vi "Add Hierarchy to Tree.vi"(7 "file name":string, 8 "error in":errorcluster, 10 "file contents":cluster{"group":string, "channels":string[]}[](array[cluster]), 11 "file tree refnum":refnum<vi>) -> (0 "error out":errorcluster)   [LabVIEW 2020, in "TdmsFileViewer.lvlib"]
uses:
  TdmsFileViewer.lvlib
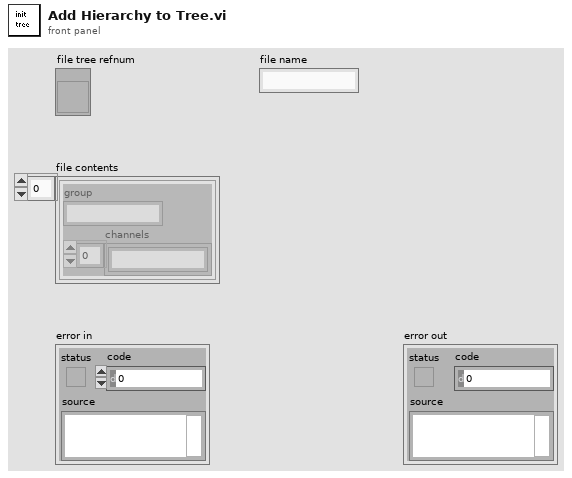
[diagram p1: front panel]
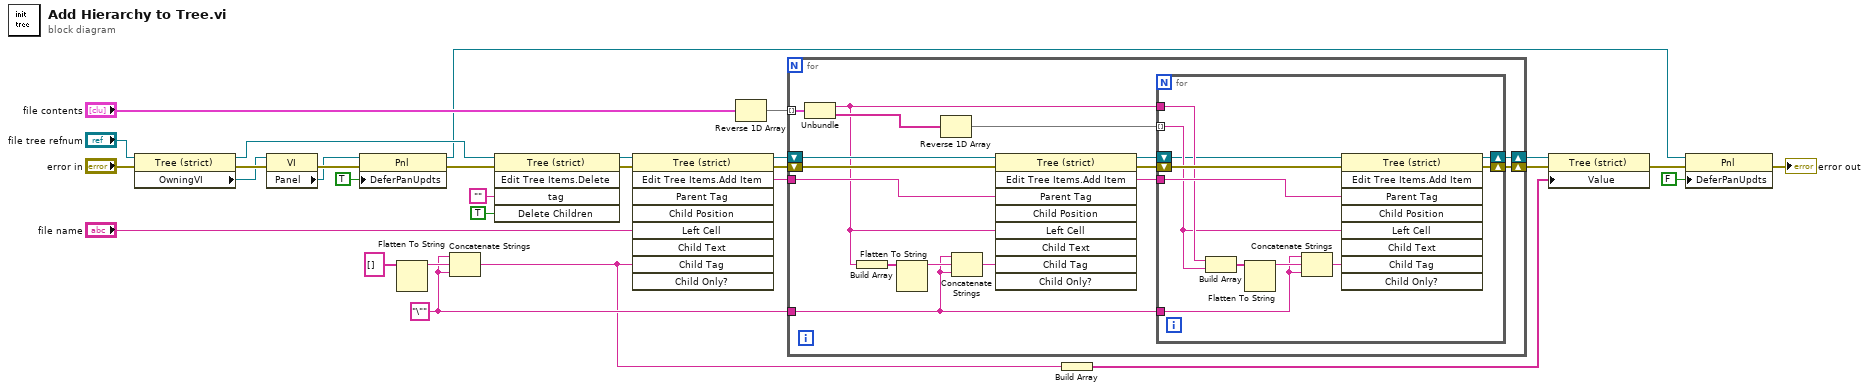
[diagram p0: block diagram]
diagram:
  w15 = "\"" ("string")
  n1 = property class="Tree (strict)"(reference="file tree refnum", error in="error in") -> (reference out=w6:refnum<vi>, error out=w26:errorcluster, "OwningVI"=w8:refnum<vi>)
  n2 = property class="VI"(reference=w8, error in=w26) -> (error out=w25:errorcluster, "Panel"=w7:refnum<vi>)  [unwired: 1 out]
  n3 = property class="Pnl"(reference=w7, error in=w25, "DeferPanUpdts"=TRUE ("Defer Panel Updates")) -> (reference out=w3:refnum<vi>, error out=w24:errorcluster)
  n4 = Flatten To String(anything=string[] [] ("appended array")) -> (data string=w18:string)  [unwired: 3 in, 2 out]
  n5 = Concatenate Strings(w15, w18, w15) -> (w2:string)
  n6 = invoke on="Invoke Node" class="Tree (strict)" method="Edit Tree Items.Delete"(reference=w6, error in=w24, "tag"="" ("Tag"), "Delete Children"=TRUE ("Delete Children?")) -> (reference out=w13:refnum<vi>, error out=w29:errorcluster)  [unwired: 1 in, 3 out]
  n7 = invoke on="Invoke Node" class="Tree (strict)" method="Edit Tree Items.Add Item"(reference=w13, error in=w29, "Left Cell"="file name", "Child Tag"=w2) -> (reference out=w20:refnum<vi>, error out=w30:errorcluster, "Edit Tree Items:Add Item"=w16:string)  [unwired: 5 in, 6 out]
  n8 = Reverse 1D Array(array="file contents") -> (reversed array=w21:cluster{"group":string, "channels":string[]}[])
  n9 = for {
    tunnel: w21 -> [w34] mode=indexing
    shift-right: [w45] -> w28
    shift-left: w30 -> [w46]
    tunnel: w16 -> [w42]
    tunnel: w15 -> [w35]
    shift-right: [w31] -> w10
    shift-left: w20 -> [w43]
    n10 = Unbundle(w34) -> ("group"=w32:string, "channels"=w33:string[])
    n11 = Build Array(w32) -> (w40:string[])
    n12 = Flatten To String(anything=w40) -> (data string=w38:string)  [unwired: 3 in, 2 out]
    n13 = Reverse 1D Array(array=w33) -> (reversed array=w39:string[])
    n14 = Concatenate Strings(w35, w38, w35) -> (w37:string)
    n15 = invoke on="Invoke Node" class="Tree (strict)" method="Edit Tree Items.Add Item"(reference=w43, error in=w46, "Parent Tag"=w42, "Left Cell"=w32, "Child Tag"=w37) -> (reference out=w36:refnum<vi>, error out=w44:errorcluster, "Edit Tree Items:Add Item"=w41:string)  [unwired: 4 in, 6 out]
    n16 = for {
      tunnel: w39 -> [w53] mode=indexing
      shift-right: [w56] -> w45
      shift-left: w44 -> [w57]
      tunnel: w41 -> [w55]
      tunnel: w32 -> [w54]
      tunnel: w35 -> [w48]
      shift-right: [w47] -> w31
      shift-left: w36 -> [w52]
      n17 = Build Array(w54, w53) -> (w51:string[])
      n18 = Flatten To String(anything=w51) -> (data string=w49:string)  [unwired: 3 in, 2 out]
      n19 = Concatenate Strings(w48, w49, w48) -> (w50:string)
      n20 = invoke on="Invoke Node" class="Tree (strict)" method="Edit Tree Items.Add Item"(reference=w52, error in=w57, "Parent Tag"=w55, "Left Cell"=w53, "Child Tag"=w50) -> (reference out=w47:refnum<vi>, error out=w56:errorcluster)  [unwired: 4 in, 7 out]
    }
  }
  n21 = Build Array(w2) -> (w1:string[])
  n22 = property class="Tree (strict)"(reference=w10, error in=w28, "Value"=w1) -> (error out=w23:errorcluster)  [unwired: 1 out]
  n23 = property class="Pnl"(reference=w3, error in=w23, "DeferPanUpdts"=FALSE ("Defer Panel Updates")) -> (error out=→"error out":errorcluster)  [unwired: 1 out]
